vi "AMC e.bloxx Tree.vi"   [LabVIEW 2013]
doc: "<B>AMC - Analytik & Messtechnik GmbH Chemnitz</B>\n\nLabVIEW Drivers for e.bloxx series from Gantner Instruments\n\nThe VI Tree displays all the user-callable VIs of the instrument driver in an organized table. It isn't executable and only for overview."
uses:
  AMC e.bloxx Write Value - Boolean.vi
  AMC e.bloxx Read Value - Boolean.vi
panel:
  # "(c) 2007 AMC - Analytik & Messtechnik Chemnitz GmbH.  ALL RIGHTS RESERVED."
  # "SEE DIAGRAM\nFOR VI TREE."
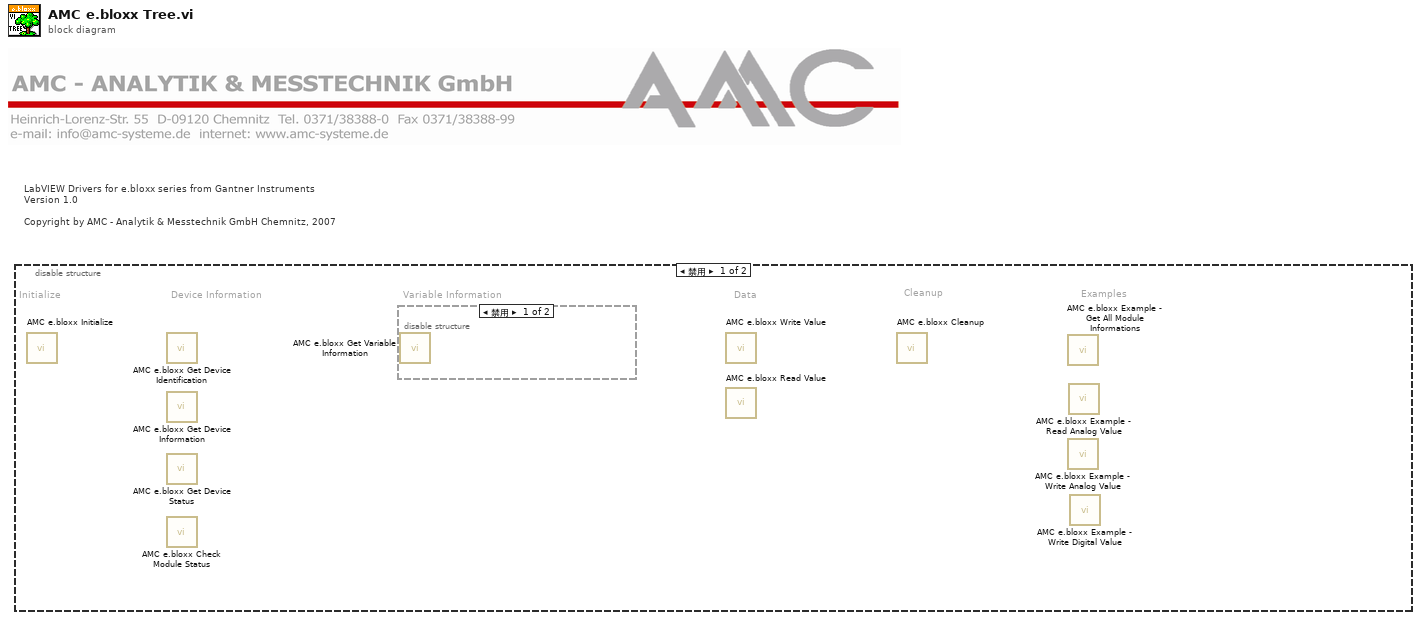
[diagram p0: block diagram]
diagram:
  # "LabVIEW Drivers for e.bloxx series from Gantner Instruments\nVersion 1.0\n\nCopyright by AMC - Analytik & Messtechnik GmbH Chemnitz, 2007"
  n1 = disable-structure shown="禁用" {
    frame Disabled {
      # "Examples"
      # "Data"
      # "Variable Information"
      # "Device Information"
      # "Cleanup"
      # "Initialize"
      n2 = call "AMC e.bloxx Initialize.vi"() -> ()  [unwired: 10 in, 2 out]
      n3 = call "AMC e.bloxx Get Device Identification.vi"() -> ()  [unwired: 6 in, 6 out]
      n4 = call "AMC e.bloxx Get Device Information.vi"() -> ()  [unwired: 7 in, 5 out]
      n5 = call "AMC e.bloxx Get Device Status.vi"() -> ()  [unwired: 8 in, 4 out]
      n6 = call "AMC e.bloxx Check Module Status.vi"() -> ()  [unwired: 9 in, 3 out]
      n7 = disable-structure shown="禁用" {
        frame Disabled {
          n8 = call "AMC e.bloxx Get Variable Information.vi"() -> ()  [unwired: 9 in, 3 out]
        }
        frame Enabled {
        }
      }
      n9 = call-poly "AMC e.bloxx Write Value.vi"() -> ()  [unwired: 10 in, 2 out]
      n10 = call-poly "AMC e.bloxx Read Value.vi"() -> ()  [unwired: 9 in, 3 out]
      n11 = call "AMC e.bloxx Cleanup.vi"() -> ()  [unwired: 11 in, 1 out]
      n12 = call "AMC e.bloxx Example - Get All Module Informations.vi"() -> ()  [unwired: 1 in]
      n13 = call "AMC e.bloxx Example - Write Analog Value.vi"() -> ()  [unwired: 1 in]
      n14 = call "AMC e.bloxx Example - Read Analog Value.vi"() -> ()  [unwired: 1 in]
      n15 = call "AMC e.bloxx Example - Write Digital Value.vi"() -> ()  [unwired: 1 in]
    }
    frame Enabled {
    }
  }
